vi "KalmanFilter01.vi"(6 "KalmanFilterVar":T1={"A"=[[1.0, 1.0], [0.0, 1.0]], "B"=[0.0, 1.0], "P0"=[[1.0, 0.0], [0.0, 1.0]], "C"=[1.0, 0.0], "Q"=[[1.0, 0.0], [0.0, 1.0]], "R"=1.0, "x0"=[0.0, 0.0]}, 10 "y":dbl, 11 "u":dbl) -> (1 "L":dbl[](array[numeric]), 2 "yhat":dbl, 3 "xhat":dbl[](array[numeric]))   [LabVIEW 2016, in "kevLib2011.lvlib"]
uses:
  kevLib2011.lvlib
  KalmanFilterVar.ctl
  <vilib>/Analysis/Matrix/Datatypes/RealMatrix.ctl
  <vilib>/Analysis/baseanly.llb/A x Vector.vi
  <vilib>/Analysis/baseanly.llb/Real Dot Product.vi
  <vilib>/Analysis/baseanly.llb/Real A x B.vi
  <vilib>/Analysis/baseanly.llb/Vector x A.vi
  <vilib>/Analysis/7linalg.llb/Real Transpose Matrix.vi
  <vilib>/Analysis/Matrix/Numeric/Subtract/Subtract - RM,RM.vi
  <vilib>/Analysis/Matrix/Numeric/Conversions/Array To Matrix - RA.vi
  <vilib>/Analysis/Matrix/Numeric/Add/Add - RM,RM.vi
  <vilib>/Analysis/7linalg.llb/Create Special Real Matrix.vi
  <vilib>/Analysis/NI_AALBase.lvlib
  <vilib>/Analysis/Matrix/NI_Matrix.lvlib
  <vilib>/Analysis/NI_AALPro.lvlib
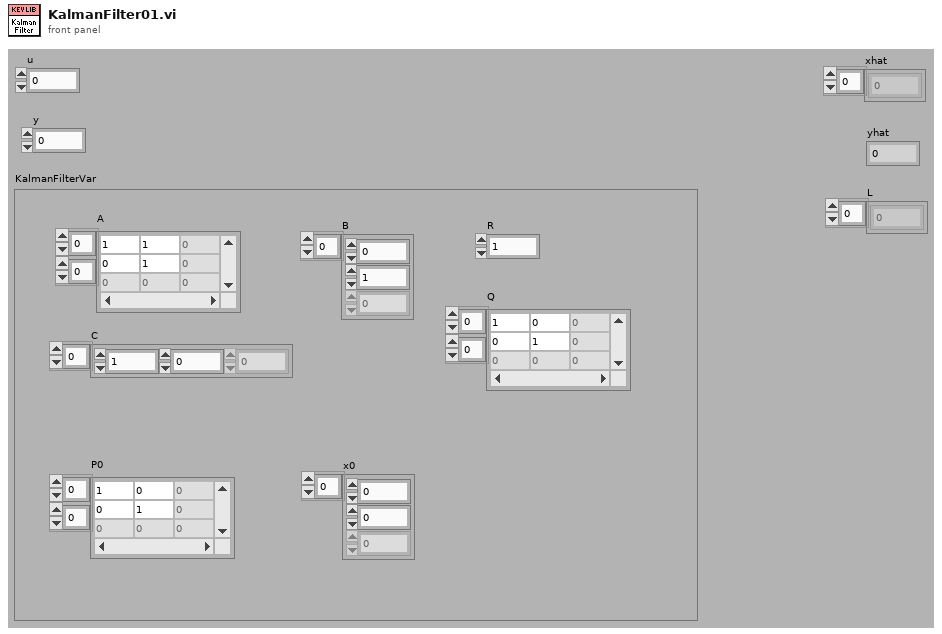
[diagram p1: front panel]
types:
  T1 = typedef "kevLib2011.lvlib/KalmanFilterVar.ctl" = cluster{"A":T2, "B":dbl[], "P0":T2, "C":dbl[], "Q":T2, "R":dbl, "x0":dbl[]}
  T2 = typedef "NI_Matrix.lvlib/RealMatrix.ctl" = dbl[][]
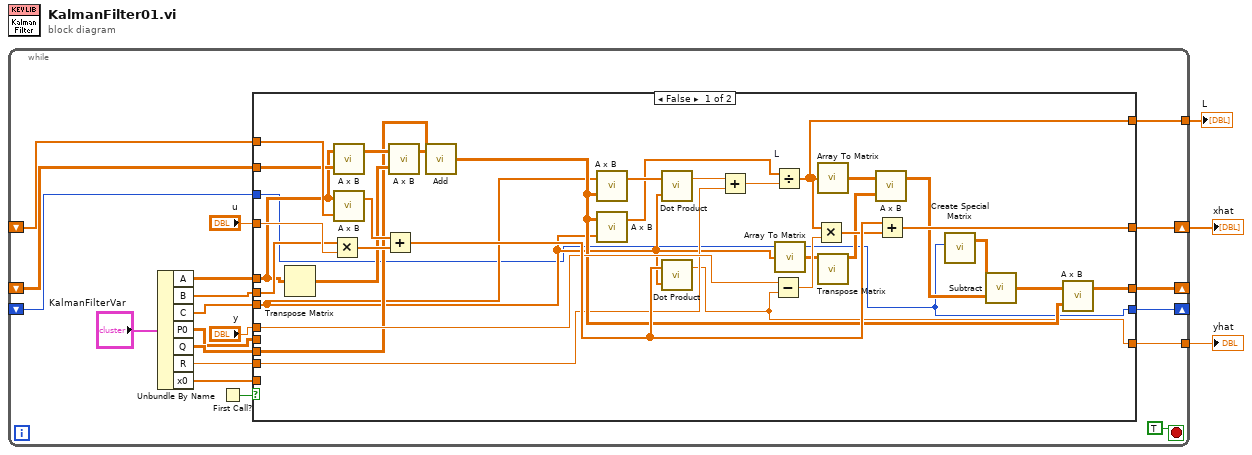
[diagram p0: block diagram]
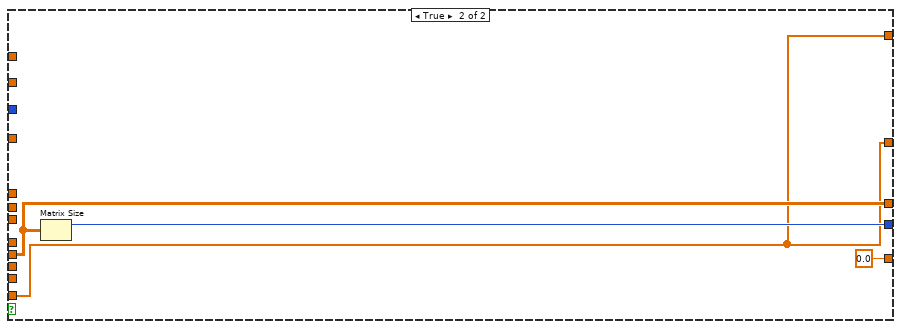
[diagram p2: hidden frame]
diagram:
  n1 = while {
    shift-right: [w22] -> w3
    shift-left: _ -> [w21]
    shift-right: [w19] -> _
    shift-left: _ -> [w18]
    shift-right: [w15] -> _
    shift-left: _ -> [w14]
    tunnel: [w5] -> w2
    tunnel: [w4] -> w1
    stop <- TRUE stop-if-true
    n2 = Unbundle By Name("KalmanFilterVar") -> ("A"=w12:T2, "B"=w11:dbl[], "C"=w6:dbl[], "P0"=w7:T2, "Q"=w10:T2, "R"=w9:dbl, "x0"=w8:dbl[])
    n3 = First Call?() -> (First Call?: T/F=w23:bool)
    n4 = case shown="False" w23 {
      tunnel: [w40 w57] -> w22
      tunnel: w21 -> [w56 _]
      tunnel: "u" -> [w55 _]
      tunnel: [w32 w59] -> w19
      tunnel: w18 -> [w52 _]
      tunnel: "y" -> [w43 _]
      tunnel: w14 -> [w26 _]
      tunnel: w10 -> [w31 _]
      tunnel: w9 -> [w30 _]
      tunnel: [w26 w60] -> w15
      tunnel: w11 -> [w29 _]
      tunnel: w12 -> [w28 _]
      tunnel: w6 -> [w27 _]
      tunnel: w7 -> [_ w59]
      tunnel: w8 -> [_ w57]
      tunnel: [w25 0.0 ("X * Y")] -> w5
      tunnel: [w24 w57] -> w4
      frame False {
        n5 = Transpose Matrix(1:w28) -> (0:w50:T2)
        n6 = Multiply(x=w29, y=w55) -> (x*y=w53:dbl[])
        n7 = call-poly <vilib>:"A x B.vi"("B"=w52, "A"=w28) -> ("A x B"=w51:T2)  [unwired: 1 out]
        n8 = call-poly <vilib>:"A x B.vi"("Vector"=w56, "A"=w28) -> ("A x Vector"=w54:dbl[])  [unwired: 1 out]
        n9 = Add(x=w54, y=w53) -> (x+y=w44:dbl[])
        n10 = call-poly <vilib>:"A x B.vi"("B"=w50, "A"=w51) -> ("A x B"=w49:T2)  [unwired: 1 out]
        n11 = call-poly <vilib>:"Add.vi"("Real Matrix B"=w31, "Real Matrix A"=w49) -> ("A + B"=w33:T2)
        n12 = call-poly <vilib>:"A x B.vi"("Matrix A"=w33, "Vector V'"=w27) -> ("V' x A"=w48:dbl[])  [unwired: 1 out]
        n13 = call-poly <vilib>:"A x B.vi"("Vector"=w27, "A"=w33) -> ("A x Vector"=w45:dbl[])  [unwired: 1 out]
        n14 = call-poly <vilib>:"Dot Product.vi"("Y Vector"=w27, "X Vector"=w48) -> ("X * Y"=w47:dbl)  [unwired: 1 out]
        n15 = call-poly <vilib>:"Dot Product.vi"("Y Vector"=w27, "X Vector"=w44) -> ("X * Y"=w25:dbl)  [unwired: 1 out]
        n16 = Add ("Add.vi")(x=w47, y=w30) -> (x+y=w46:dbl)
        n17 = Subtract(x=w43, y=w25) -> (x-y=w42:dbl)
        n18 = Divide "L"(x=w45, y=w46) -> (x/y=w24:dbl[])
        n19 = call-poly <vilib>:"Array To Matrix.vi"("Real 1D Array"=w27) -> ("Real Matrix (Column Vector)"=w39:T2)
        n20 = Multiply ("Multiply.vi")(x=w24, y=w42) -> (x*y=w41:dbl[])
        n21 = call-poly <vilib>:"Array To Matrix.vi"("Real 1D Array"=w24) -> ("Real Matrix (Column Vector)"=w36:T2)
        n22 = call-poly <vilib>:"Transpose Matrix.vi"("Input Matrix"=w39) -> ("Matrix Transpose"=w38:T2)  [unwired: 9 in, 1 out]
        n23 = call-poly <vilib>:"A x B.vi"("B"=w38, "A"=w36) -> ("A x B"=w37:T2)  [unwired: 1 out]
        n24 = Add ("Add.vi")(x=w44, y=w41) -> (x+y=w40:dbl[])
        n25 = call-poly <vilib>:"Create Special Matrix.vi"("matrix size"=w26) -> ("Special Matrix"=w35:T2)  [unwired: 4 in, 1 out]
        n26 = call-poly <vilib>:"Subtract.vi"("Real Matrix B"=w37, "Real Matrix A"=w35) -> ("A - B"=w34:T2)
        n27 = call-poly <vilib>:"A x B.vi"("B"=w33, "A"=w34) -> ("A x B"=w32:T2)  [unwired: 1 out]
      }
      frame True {
        n28 = Matrix Size(0:w59) -> (1:w60:i32)  [unwired: 1 out]
      }
    }
  }
  "xhat" <- w3
  "yhat" <- w2
  "L" <- w1
